vi "SBML_Species_Parser.vi"(8 "error in (no error)":errorcluster, 11 "Input SBML File":string) -> (0 "error out":errorcluster, 1 "Species Info":string[][](array[string]), 3 "Sp_Cnt":i32)   [LabVIEW 2014]
doc: "This VI extract the information of species present in SBML file. It takes the complete SBML file as input, and outputs: \nSp_Cnt --> How many species are there\nS_Id_Arr --> Array of species\nSp_Name --> Array containing the name of species\nSp_Init_Amnt --> Array containing the initial amount of species\n\nDesigned by HB\nhaba@dtu.dk"
panel:
  out "Constant":string[](array[string])
  out "Conversion Factor":string[](array[string])
  out "Boundary Conditions":string[](array[string])
  out "Only Substance Units":string[](array[string])
  out "Units":string[](array[string])
  out "Init Concentration":string[](array[string])
  out "Compartment":string[](array[string])
  out "Order":string[](array[string])
  out "Sp_Init_Amnt":string[](array[string])
  out "Sp_Name":string[](array[string])
  out "Sp_Id_Arr":string[](array[string])
  out "List of Species":string
  # "Only Susbtance\nUnits"
  # "Initial \nConcentration"
  # "Boundary\nCondition"
  # "Initial \nAmount"
  # "Conversion\nFactor"
  # "Constant"
  # "Compartment"
  # "Units"
  # "ID"
  # "Name"
  # "Names"
  # "Initial Amount"
  # "ID"
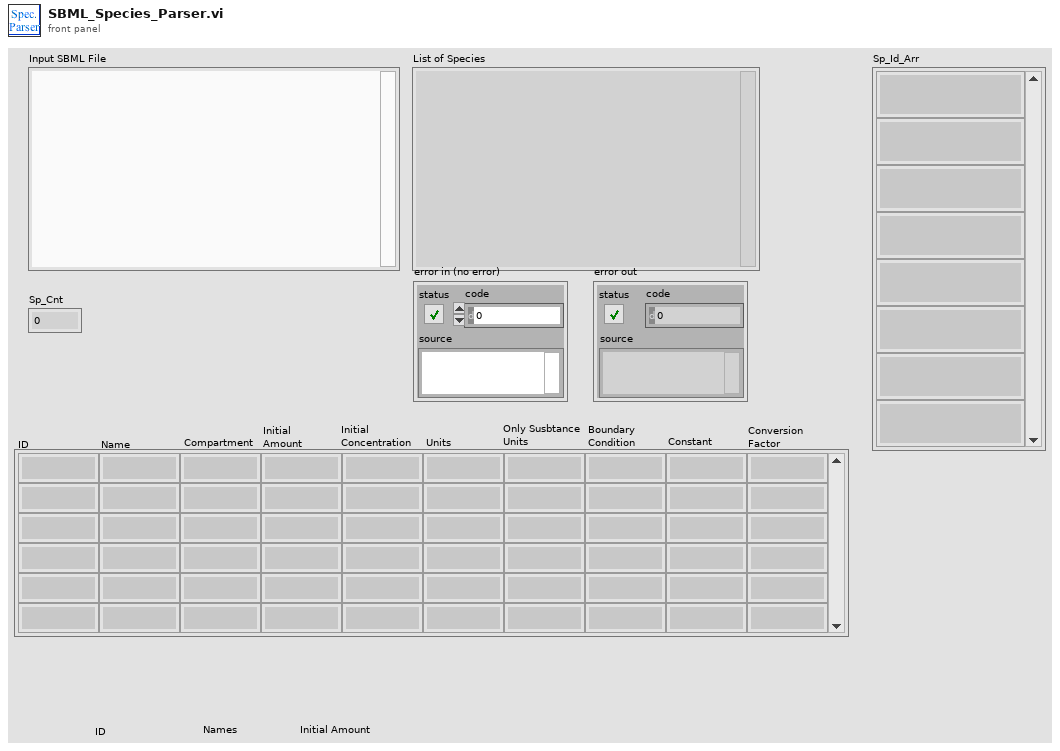
[diagram p1: front panel]
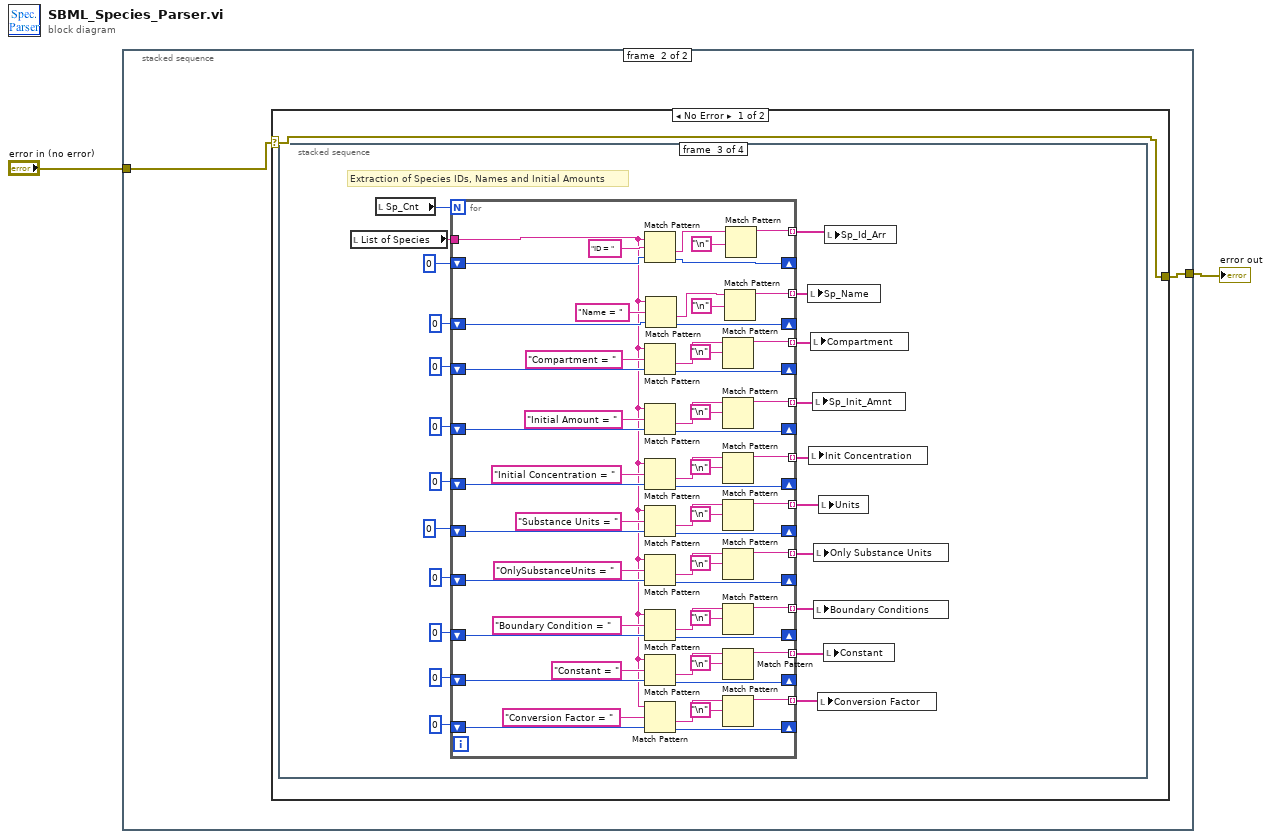
[diagram p0: block diagram]
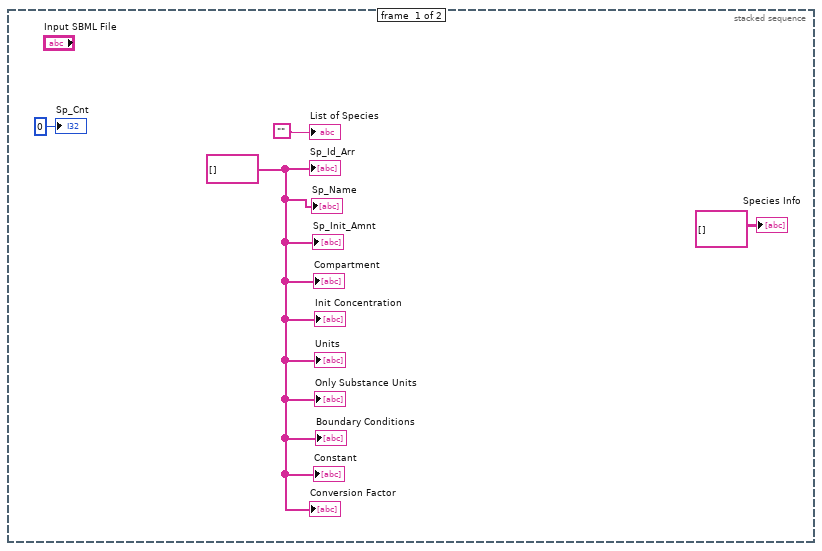
[diagram p2: hidden frame]
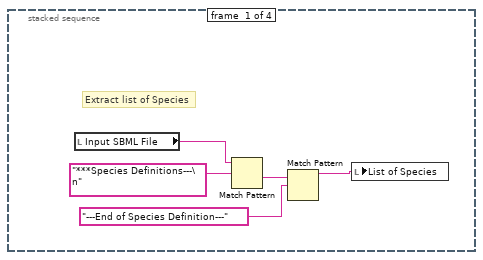
[diagram p3: hidden frame]
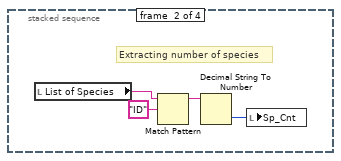
[diagram p4: hidden frame]
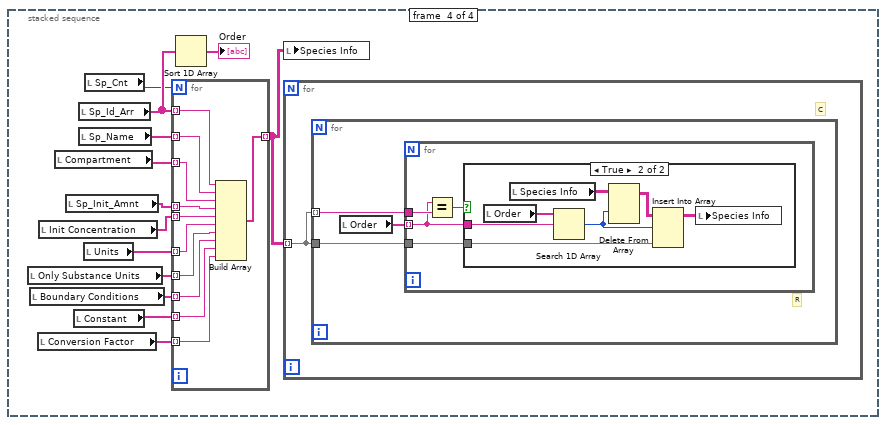
[diagram p5: hidden frame]
diagram:
  n1 = stacked-sequence {
    tunnel: "error in (no error)" -> [_ w7]
    tunnel: [_ w8] -> w1
    frame #0 {
      w3 = string[] [] ("Sp_Id_Arr")
      "List of Species" <- "" ("Full SBML File")
      "Sp_Cnt" <- 0 ("Sp_cnt")
      "Sp_Id_Arr" <- w3
      "Sp_Name" <- w3
      "Sp_Init_Amnt" <- w3
      "Species Info" <- string[][] [] ("Species Info")
      "Compartment" <- w3
      "Init Concentration" <- w3
      "Units" <- w3
      "Only Substance Units" <- w3
      "Boundary Conditions" <- w3
      "Conversion Factor" <- w3
      "Constant" <- w3
    }
    frame #1 {
      n2 = case shown="No Error" w7 {
        selector: w7 -> [w9 w141]
        tunnel: [w9 w141] -> w8
        frame No Error {
          n3 = stacked-sequence {
            frame #0 {
              # "Extract list of Species"
              n4 = local read "Input SBML File"() -> (w11:string)
              n5 = Match Pattern(string=w11, regular expression="***Species Definitions---\n") -> (after substring=w13:string)  [unwired: 1 in, 3 out]
              n6 = Match Pattern(string=w13, regular expression="---End of Species Definition---") -> (before substring=w10:string)  [unwired: 1 in, 3 out]
              n7 = local write "List of Species"(w10) -> ()
            }
            frame #1 {
              # "Extracting number of species"
              n8 = local read "List of Species"() -> (w15:string)
              n9 = Match Pattern(string=w15, regular expression="ID") -> (before substring=w17:string)  [unwired: 1 in, 3 out]
              n10 = Decimal String To Number(string=w17) -> (number=w16:i32)  [unwired: 2 in, 1 out]
              n11 = local write "Sp_Cnt"(w16) -> ()
            }
            frame #2 {
              # "Extraction of Species IDs, Names and Initial Amounts"
              n12 = local read "List of Species"() -> (w36:string)
              n13 = local read "Sp_Cnt"() -> (w35:i32)
              n14 = for {
                N: w35 -> [_]
                tunnel: w36 -> [w41]
                shift-right: [w97] -> _
                shift-left: 0 ("offset of match") -> [w96]
                tunnel: [w98] -> w38 mode=indexing
                shift-right: [w92] -> _
                shift-left: 0 ("offset past match") -> [w91]
                shift-right: [w87] -> _
                shift-left: 0 ("offset past match") -> [w86]
                tunnel: [w85] -> w34 mode=indexing
                tunnel: [w84] -> w33 mode=indexing
                shift-right: [w82] -> _
                shift-left: 0 ("offset of match") -> [w83]
                tunnel: [w81] -> w31 mode=indexing
                shift-right: [w73] -> _
                shift-left: 0 ("offset of match") -> [w72]
                tunnel: [w74] -> w30 mode=indexing
                shift-right: [w70] -> _
                shift-left: 0 ("offset of match") -> [w71]
                tunnel: [w69] -> w27 mode=indexing
                shift-right: [w61] -> _
                shift-left: 0 ("offset of match") -> [w60]
                tunnel: [w62] -> w26 mode=indexing
                shift-right: [w58] -> _
                shift-left: 0 ("offset of match") -> [w59]
                tunnel: [w57] -> w23 mode=indexing
                shift-right: [w49] -> _
                shift-left: 0 ("offset of match") -> [w48]
                tunnel: [w50] -> w22 mode=indexing
                shift-right: [w46] -> _
                shift-left: 0 ("offset of match") -> [w47]
                tunnel: [w45] -> w19 mode=indexing
                n15 = Match Pattern(string=w41, regular expression="ID = ", offset (0)=w86) -> (after substring=w88:string, offset past match=w87:i32)  [unwired: 2 out]
                n16 = Match Pattern(string=w41, regular expression="Compartment = ", offset (0)=w96) -> (after substring=w99:string, offset past match=w97:i32)  [unwired: 2 out]
                n17 = Match Pattern(string=w41, regular expression="Initial Amount = ", offset (0)=w83) -> (after substring=w80:string, offset past match=w82:i32)  [unwired: 2 out]
                n18 = Match Pattern(string=w41, regular expression="Initial Concentration = ", offset (0)=w72) -> (after substring=w75:string, offset past match=w73:i32)  [unwired: 2 out]
                n19 = Match Pattern(string=w41, regular expression="Substance Units = ", offset (0)=w71) -> (after substring=w68:string, offset past match=w70:i32)  [unwired: 2 out]
                n20 = Match Pattern(string=w41, regular expression="OnlySubstanceUnits = ", offset (0)=w60) -> (after substring=w63:string, offset past match=w61:i32)  [unwired: 2 out]
                n21 = Match Pattern(string=w41, regular expression="Boundary Condition = ", offset (0)=w59) -> (after substring=w56:string, offset past match=w58:i32)  [unwired: 2 out]
                n22 = Match Pattern(string=w41, regular expression="Constant = ", offset (0)=w48) -> (after substring=w51:string, offset past match=w49:i32)  [unwired: 2 out]
                n23 = Match Pattern(string=w41, regular expression="Conversion Factor = ", offset (0)=w47) -> (after substring=w44:string, offset past match=w46:i32)  [unwired: 2 out]
                n24 = Match Pattern(string=w41, regular expression="Name = ", offset (0)=w91) -> (after substring=w95:string, offset past match=w92:i32)  [unwired: 2 out]
                n25 = Match Pattern(string=w99, regular expression="\n") -> (before substring=w98:string)  [unwired: 1 in, 3 out]
                n26 = Match Pattern(string=w80, regular expression="\n") -> (before substring=w81:string)  [unwired: 1 in, 3 out]
                n27 = Match Pattern(string=w75, regular expression="\n") -> (before substring=w74:string)  [unwired: 1 in, 3 out]
                n28 = Match Pattern(string=w68, regular expression="\n") -> (before substring=w69:string)  [unwired: 1 in, 3 out]
                n29 = Match Pattern(string=w63, regular expression="\n") -> (before substring=w62:string)  [unwired: 1 in, 3 out]
                n30 = Match Pattern(string=w56, regular expression="\n") -> (before substring=w57:string)  [unwired: 1 in, 3 out]
                n31 = Match Pattern(string=w51, regular expression="\n") -> (before substring=w50:string)  [unwired: 1 in, 3 out]
                n32 = Match Pattern(string=w44, regular expression="\n") -> (before substring=w45:string)  [unwired: 1 in, 3 out]
                n33 = Match Pattern(string=w95, regular expression="\n") -> (before substring=w85:string)  [unwired: 1 in, 3 out]
                n34 = Match Pattern(string=w88, regular expression="\n") -> (before substring=w84:string)  [unwired: 1 in, 3 out]
              }
              n35 = local write "Sp_Name"(w34) -> ()
              n36 = local write "Init Concentration"(w30) -> ()
              n37 = local write "Compartment"(w38) -> ()
              n38 = local write "Sp_Init_Amnt"(w31) -> ()
              n39 = local write "Only Substance Units"(w26) -> ()
              n40 = local write "Boundary Conditions"(w23) -> ()
              n41 = local write "Conversion Factor"(w19) -> ()
              n42 = local write "Units"(w27) -> ()
              n43 = local write "Constant"(w22) -> ()
              n44 = local write "Sp_Id_Arr"(w33) -> ()
            }
            frame #3 {
              n45 = local read "Only Substance Units"() -> (w105:string[])
              n46 = local read "Boundary Conditions"() -> (w104:string[])
              n47 = local read "Conversion Factor"() -> (w102:string[])
              n48 = local read "Init Concentration"() -> (w107:string[])
              n49 = local read "Compartment"() -> (w112:string[])
              n50 = local read "Sp_Init_Amnt"() -> (w108:string[])
              n51 = local read "Constant"() -> (w103:string[])
              n52 = local read "Sp_Id_Arr"() -> (w113:string[])
              n53 = local read "Sp_Name"() -> (w111:string[])
              n54 = local read "Units"() -> (w106:string[])
              n55 = local read "Sp_Cnt"() -> (w110:i32)
              n56 = for {
                N: w110 -> [_]
                tunnel: w113 -> [w140] mode=indexing
                tunnel: w111 -> [w139] mode=indexing
                tunnel: w112 -> [w138] mode=indexing
                tunnel: [w137] -> w109 mode=indexing
                tunnel: w108 -> [w136] mode=indexing
                tunnel: w107 -> [w135] mode=indexing
                tunnel: w106 -> [w134] mode=indexing
                tunnel: w105 -> [w133] mode=indexing
                tunnel: w104 -> [w132] mode=indexing
                tunnel: w103 -> [w131] mode=indexing
                tunnel: w102 -> [w130] mode=indexing
                n57 = Build Array(w140, w139, w138, w136, w135, w134, w133, w132, w131, w130) -> (w137:string[])
              }
              n58 = Sort 1D Array(array=w113) -> (sorted array=→"Order":string[])
              n59 = local write "Species Info"(w109) -> ()
              n60 = for {
                tunnel: w109 -> [w115] mode=indexing
                # "C"
                n61 = for {
                  tunnel: w115 -> [w117] mode=indexing
                  tunnel: w115 -> [w116]
                  # "R"
                  n62 = local read "Order"() -> (w118:string[])
                  n63 = for {
                    tunnel: w118 -> [w120] mode=indexing
                    tunnel: w117 -> [w122]
                    tunnel: w116 -> [w119]
                    n64 = Equal?(x=w120, y=w122) -> (x = y?=w121:bool)
                    n65 = case shown="True" w121 {
                      tunnel: w120 -> [_ w128]
                      tunnel: w119 -> [_ w127]
                      frame False {
                      }
                      frame True {
                        n66 = local read "Order"() -> (w129:string[])
                        n67 = local read "Species Info"() -> (w125:string[][])
                        n68 = Search 1D Array(1D array=w129, element=w128) -> (index of element=w124:i32)  [unwired: 1 in]
                        n69 = Delete From Array(array=w125, index (row)=w124) -> (array with subset deleted=w123:string[][])  [unwired: 2 in, 1 out]
                        n70 = Insert Into Array(array=w123, index (row)=w124, new element=w127) -> (w126:string[][])  [unwired: 1 in]
                        n71 = local write "Species Info"(w126) -> ()
                      }
                    }
                  }
                }
              }
            }
          }
        }
        frame Error {
        }
      }
    }
  }
  "error out" <- w1
